vi "AUTORESAMPLE(SubVI).vi"(8 "Error In":errorcluster, 9 "Y Resolution":i32, 10 "X Resolution":i32, 11 "Image In":T1) -> (0 "Error Out":errorcluster, 3 "Image Resize Out":T1)   [LabVIEW 2011]
doc: "Se autoresample a una X e Y resolution determinada."
uses:
  IMAQ Image.ctl
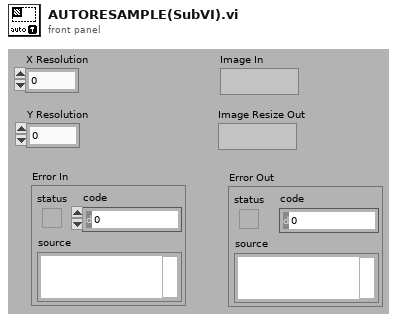
[diagram p1: front panel]
types:
  T1 = typedef "IMAQ Image.ctl" = cluster{string, u32}
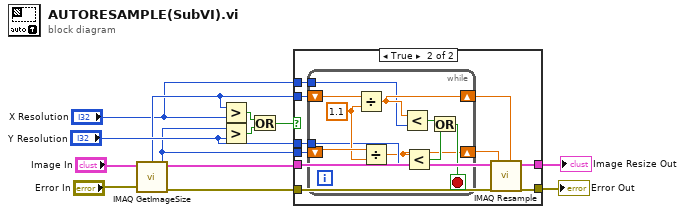
[diagram p0: block diagram]
diagram:
  n1 = call "IMAQ GetImageSize"("Image"="Image In", "error in (no error)"="Error In") -> ("Y Resolution"=w8:i32, "X Resolution"=w7:i32, "error out"=w2:errorcluster)  [unwired: 2 out]
  n2 = Greater?(x=w7, y="X Resolution") -> (0:w5:bool)
  n3 = Greater?(x=w8, y="Y Resolution") -> (0:w6:bool)
  n4 = Or(x=w5, y=w6) -> (x .or. y?=w4:bool)
  n5 = case shown="True" w4 {
    tunnel: w7 -> [_ w18]
    tunnel: "Image In" -> [w14 w24]
    tunnel: w2 -> [w13 w23]
    tunnel: [w13 w22] -> w9
    tunnel: [w14 w21] -> w3
    tunnel: w8 -> [_ w17]
    tunnel: "Y Resolution" -> [_ w16]
    tunnel: "X Resolution" -> [_ w15]
    frame False {
    }
    frame True {
      n6 = while {
        shift-right: [w25] -> w20
        shift-left: w17 -> [w34]
        shift-right: [w33] -> w19
        shift-left: w18 -> [w32]
        tunnel: w16 -> [w27]
        tunnel: w15 -> [w26]
        stop <- w29 stop-if-true
        w28 = 1.1 ("y")
        n7 = Divide(x=w32, y=w28) -> (x/y=w33:dbl)
        n8 = Divide(x=w34, y=w28) -> (x/y=w25:dbl)
        n9 = Less?(x=w33, y=w26) -> (x < y?=w31:bool)
        n10 = Less?(x=w25, y=w27) -> (x < y?=w30:bool)
        n11 = Or(x=w31, y=w30) -> (x .or. y?=w29:bool)
      }
      n12 = call "IMAQ Resample"("X Resolution"=w19, "Y Resolution"=w20, "error in (no error)"=w23, "Image Src"=w24) -> ("error out"=w22:errorcluster, "Image Dst Out"=w21:T1)  [unwired: 3 in, 3 out]
    }
  }
  "Error Out" <- w9
  "Image Resize Out" <- w3
